vi "Build Tx UDP Engine Configuration.vi"(0 "section ref in":T8=18446744073709551615 format="%.0x", 5 "board properties":T6 {"portConfig" items=["FDX_SINGLE", "FDX_REDUNDANT"]; "portSpeed" items=["FDX_100MBIT", "FDX_10MBIT", "FDX_AUTO_100MBIT", "FDX_AUTO_10MBIT", "FDX_AUTO_ERROR", "FDX_1000MBIT"]}, 9 "port properties":T5, 11 "error in":errorcluster) -> (4 "section ref out":T8 format="%.0x", 6 "boardId":u32, 8 "portId":u32, 10 "VL configurations":T7(array[cluster]) {"VL Config"."NetSelect" items=["FDX_TX_FRAME_DLY_A"=0, "FDX_TX_FRAME_DLY_B"=1, "FDX_TX_FRAME_BOTH "=3, "FDX_TX_FRAME_ONLY_A"=4, "FDX_TX_FRAME_ONLY_B "=5]; "VL Config"."interfaceID" format="%.0b"}, 14 "comm port payload":T4(array[cluster]), 15 "error out":errorcluster)   [LabVIEW 2020, in "AIM ARINC 664 Scripting.lvlib"]
uses:
  AIM ARINC 664 Scripting.lvlib
  <vilib>/NI VeriStand/Custom Device API/Custom Device Item Ref.ctl
  <instrlib>/AIM GmbH/_AIM 664/_controls/comm_config_vl_tx.ctl
  <instrlib>/AIM GmbH/_AIM 664/_controls/comm_udp_tx.ctl
  Shared/board_setup.ctl
  Shared/port_setup.ctl
  <vilib>/NI/NI VeriStand Encoding and Decoding/Encoding.ctl
  <instrlib>/AIM GmbH/_AIM 664/AIM664LV.lvlib
  <vilib>/NI VeriStand/Custom Device API/Custom Device API.lvlib
  <vilib>/NI/NI VeriStand Encoding and Decoding/Encoding and Decoding.lvlib
  <vilib>/Utility/SystemLogging/NI_SystemLogging.lvlib
  Import/AIM ARINC 664 Import.lvlib
panel:
  in  "Cluster":cluster{"VL Config":T1, "CommPort Config":T2[]} {"VL Config"."NetSelect" items=["FDX_TX_FRAME_DLY_A"=0, "FDX_TX_FRAME_DLY_B"=1, "FDX_TX_FRAME_BOTH "=3, "FDX_TX_FRAME_ONLY_A"=4, "FDX_TX_FRAME_ONLY_B "=5]; "VL Config"."interfaceID" format="%.0b"}
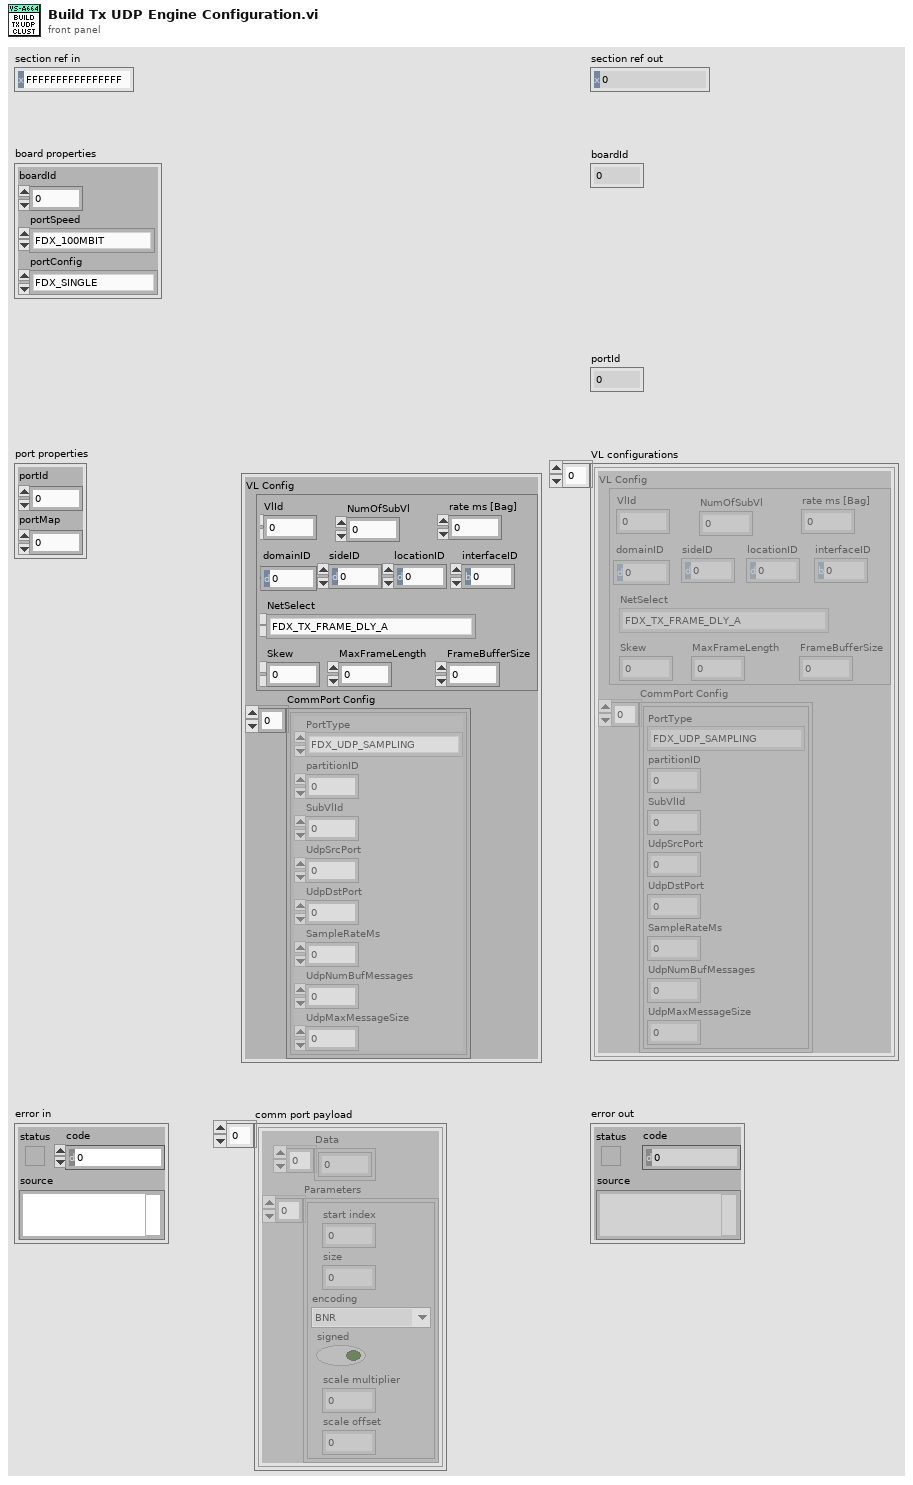
[diagram p1: front panel]
types:
  T1 = typedef "AIM664LV.lvlib/comm_config_vl_tx.ctl" = cluster{"VlId":u16, "NumOfSubVl":u16, "rate ms [Bag]":u32, "domainID":u8, "sideID":u8, "locationID":u8, "interfaceID":u8, "NetSelect":u32, "Skew":u32, "MaxFrameLength":u32, "FrameBufferSize":u32}
  T2 = typedef "AIM664LV.lvlib/comm_udp_tx.ctl" = cluster{"PortType":enum16{"FDX_UDP_SAMPLING", "FDX_UDP_QUEUING"}, "partitionID":u8, "SubVlId":u8, "UdpSrcPort":u16, "UdpDstPort":u16, "SampleRateMs":dbl, "UdpNumBufMessages":u32, "UdpMaxMessageSize":u32}
  T3 = typedef "Encoding and Decoding.lvlib/Encoding.ctl" = enum16{"BNR", "BCD", "Discrete"}
  T4 = cluster{"Data":u8[], "Parameters":cluster{"start index":i32, "size":i32, "encoding":T3, "signed":bool, "scale multiplier":dbl, "scale offset":dbl}[]}[]
  T5 = typedef "AIM ARINC 664 Import.lvlib/port_setup.ctl" = cluster{"portId":u32, "portMap":u32}
  T6 = typedef "AIM ARINC 664 Import.lvlib/board_setup.ctl" = cluster{"boardId":u32, "portSpeed":u32, "portConfig":u32}
  T7 = cluster{"VL Config":T1, "CommPort Config":T2[]}[]
  T8 = typedef "Custom Device API.lvlib/Custom Device Item Ref.ctl" = u64
  T9 = cluster{"Data":u8[], "Parameters":cluster{"start index":i32, "size":i32, "encoding":T3, "signed":bool, "scale multiplier":dbl, "scale offset":dbl}[]}
  T10 = cluster{"start index":i32, "size":i32, "encoding":T3, "signed":bool, "scale multiplier":dbl, "scale offset":dbl}
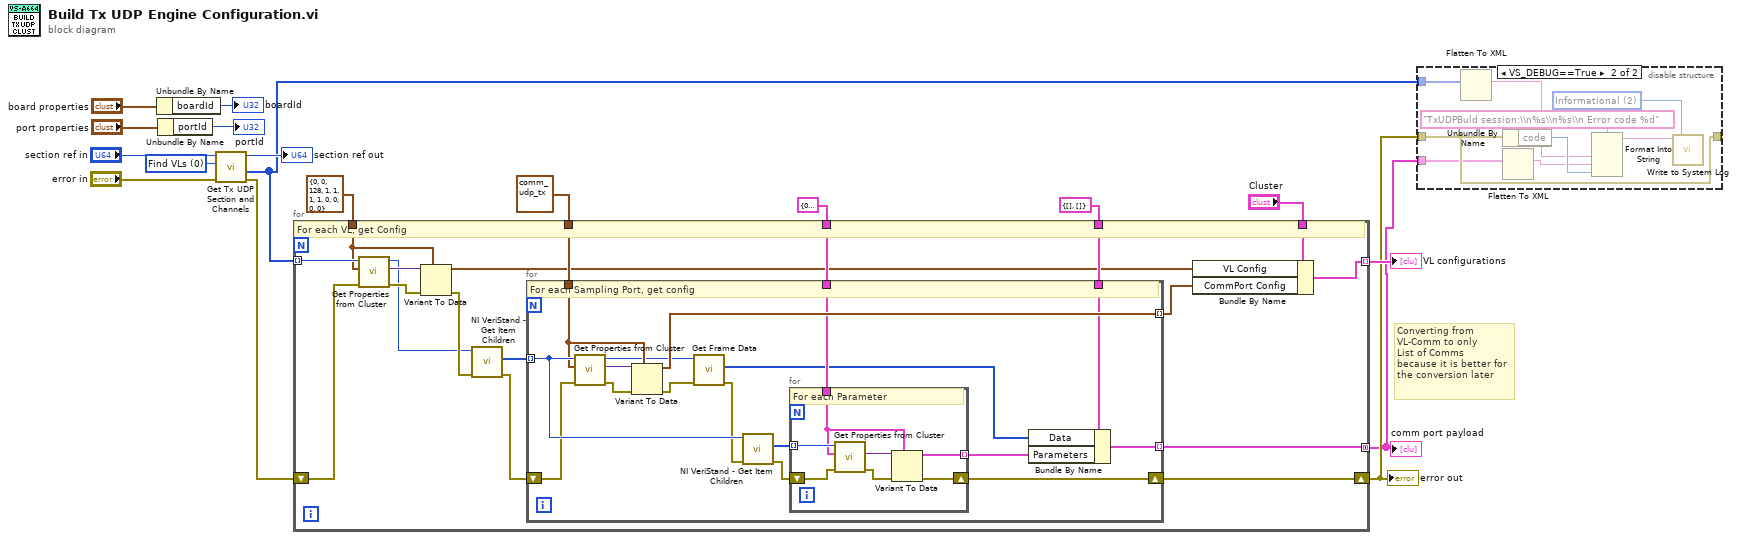
[diagram p0: block diagram]
diagram:
  w13 = u16 0 items=["Find VLs", "Find Parameters"] ("Option")
  # "Converting from \nVL-Comm to only\nList of Comms\nbecause it is better for\nthe conversion later"
  n1 = Unbundle By Name("board properties") -> ("boardId"=→"boardId":u32)
  n2 = Unbundle By Name("port properties") -> ("portId"=→"portId":u32)
  n3 = call "Get Tx UDP Section and Channels.vi"("error in"="error in", "option"=w13, "custom device ref in"="section ref in") -> ("error out"=w9:errorcluster, "Tx UDP channel refs out"=w3:T8[], "custom device ref out"=→"section ref out":T8)  [unwired: 3 in, 3 out]
  n4 = for {
    tunnel: [w27] -> w16 mode=indexing
    tunnel: w3 -> [w36] mode=indexing
    tunnel: T1 {"VlId"=0, "NumOfSubVl"=0, "rate ms [Bag]"=128, "domainID"=1, "sideID"=1, "locationID"=1, "interfaceID"=1, "NetSelect"=0, "Skew"=0, "MaxFrameLength"=0, "FrameBufferSize"=0} ("CommPort Config") -> [w34]
    shift-right: [w21] -> w4
    shift-left: w9 -> [w35]
    tunnel: T2 {"PortType"=enum."FDX_UDP_SAMPLING", "partitionID"=0, "SubVlId"=1, "UdpSrcPort"=0, "UdpDstPort"=0, "SampleRateMs"=128.0, "UdpNumBufMessages"=0, "UdpMaxMessageSize"=0} ("commPort config") -> [w26]
    tunnel: T10 {"start index"=0, "size"=0, "encoding"=enum."BNR", "signed"=FALSE, "scale multiplier"=0.0, "scale offset"=0.0} ("Parameter") -> [w24]
    tunnel: [w22] -> w1 mode=concatenating
    tunnel: T9 {"Data"=[], "Parameters"=[]} ("Data and Parameters") -> [w23]
    tunnel: "Cluster" -> [w19]
    # "For each VL, get Config"
    n5 = call "Get Properties from Cluster.vi"("error in"=w35, "Variant Cluster"=w34, "custom device ref in"=w36) -> ("error out"=w32:errorcluster, "data"=w33:variant, "custom device ref out"=w30:T8)  [unwired: 5 in, 1 out]
    n6 = Variant To Data(error in=w32, type=w34, Variant=w33) -> (data=w20:T1, error out=w31:errorcluster)
    n7 = call <vilib>:"NI VeriStand - Get Item Children.vi"("error in (no error)"=w31, "Item Ref in"=w30) -> ("error out"=w28:errorcluster, "Child Refs"=w29:T8[])  [unwired: 6 in, 2 out]
    n8 = for {
      tunnel: w29 -> [w49] mode=indexing
      shift-right: [w42] -> w21
      shift-left: w28 -> [w41]
      tunnel: w26 -> [w48]
      tunnel: [w47] -> w25 mode=indexing
      tunnel: w24 -> [w46]
      tunnel: w23 -> [w45]
      tunnel: [w43] -> w22 mode=indexing
      # "For each Sampling Port, get config"
      n9 = call "Get Properties from Cluster.vi"("error in"=w41, "Variant Cluster"=w48, "custom device ref in"=w49) -> ("error out"=w51:errorcluster, "data"=w50:variant, "custom device ref out"=w40:T8)  [unwired: 5 in, 1 out]
      n10 = Variant To Data(error in=w51, type=w48, Variant=w50) -> (data=w47:T2, error out=w39:errorcluster)
      n11 = call "Get Frame Data.vi"("error in"=w39, "Frame Ref"=w40) -> ("error out"=w38:errorcluster, "Data"=w37:u8[])  [unwired: 7 in, 1 out]
      n12 = call <vilib>:"NI VeriStand - Get Item Children.vi"("error in (no error)"=w38, "Item Ref in"=w49) -> ("error out"=w52:errorcluster, "Child Refs"=w53:T8[])  [unwired: 6 in, 2 out]
      n13 = for {
        tunnel: w53 -> [w58] mode=indexing
        shift-right: [w54] -> w42
        shift-left: w52 -> [w55]
        tunnel: w46 -> [w57]
        tunnel: [w56] -> w44 mode=indexing
        # "For each Parameter"
        n14 = call "Get Properties from Cluster.vi"("error in"=w55, "Variant Cluster"=w57, "custom device ref in"=w58) -> ("error out"=w59:errorcluster, "data"=w60:variant)  [unwired: 5 in, 2 out]
        n15 = Variant To Data(error in=w59, type=w57, Variant=w60) -> (data=w56:T10, error out=w54:errorcluster)
      }
      n16 = Bundle By Name(cluster=w45, "Data"=w37, "Parameters"=w44) -> (w43:T9)
    }
    n17 = Bundle By Name(cluster=w19, "VL Config"=w20, "CommPort Config"=w25) -> (w27:cluster{"VL Config":T1, "CommPort Config":T2[]})
  }
  "error out" <- w4
  "VL configurations" <- w16
  "comm port payload" <- w1
  n18 = disable-structure shown="VS_DEBUG==True" {
    disable-tunnel: w4 -> [_ w65]
    disable-tunnel: [_ w65] -> _
    disable-tunnel: w1 -> [_ w64]
    disable-tunnel: w3 -> [_ w61]
    frame condition #0 (active) {
    }
    frame condition #1 {
      w67 = 2 items=["Error", "Warning", "Informational"] ("severity")
      n19 = Flatten To XML(6:w61) -> (2:w62:string)
      n20 = Unbundle By Name(w65) -> ("code"=w66:i32)
      n21 = Flatten To XML(6:w64) -> (2:w63:string)
      n22 = Format Into String(format string="TxUDPBuld session:\\n%s\\n%s\\n Error code %d", w62, w63, w66) -> (resulting string=w68:string)  [unwired: 2 in, 1 out]
      n23 = call <vilib>:"Write to System Log.vi"("severity"=w67, "message"=w68) -> ()  [unwired: 9 in, 1 out]
    }
  }
